vi "Set Window Titel.vi"(8 "error in (no error)":errorcluster, 10 "Title":string, 11 "ViewableActor in":refnum<class "ViewableActor.lvclass">) -> (0 "error out":errorcluster, 3 "ViewableActor out":refnum<class "ViewableActor.lvclass">)   [LabVIEW 2020, in "ViewableActor.lvlib" / "ViewableActor.lvclass"]
uses:
  ViewableActor.lvclass
  ViewableActor.lvclass/ViewableActor.ctl
  Read UI VI Ref.vi
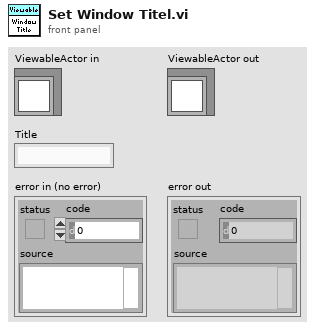
[diagram p1: front panel]
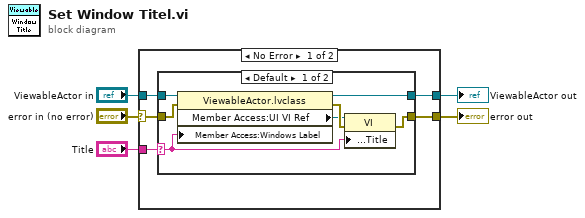
[diagram p0: block diagram]
diagram:
  n1 = case shown="No Error" "error in (no error)" {
    selector: "error in (no error)" -> [w7 w21]
    tunnel: [w8 w21] -> w4
    tunnel: [w9 w20] -> w2
    tunnel: "ViewableActor in" -> [w10 w20]
    tunnel: "Title" -> [w6 _]
    frame No Error {
      n2 = case shown="Default" w6 {
        selector: w6 -> [w11 _]
        tunnel: [w17 w18] -> w8
        tunnel: w10 -> [w16 w19]
        tunnel: [w15 w19] -> w9
        tunnel: w7 -> [w14 w18]
        frame Default {
          n3 = property class="ViewableActor.lvclass"(reference=w16, error in=w14, "Member Access:Windows Label"=w11) -> (reference out=w15:refnum<class "ViewableActor.lvclass">, error out=w13:errorcluster, "Member Access:UI VI Ref"=w12:refnum<vi>)
          n4 = property class="VI"(reference=w12, error in=w13, "Front Panel.Title"=w11) -> (error out=w17:errorcluster)  [unwired: 1 out]
        }
        frame "" {
        }
      }
    }
    frame Error {
    }
  }
  "error out" <- w4
  "ViewableActor out" <- w2
